vi "serial_connection_FSM_2.vi"(0 "commands_q":refnum<queue>, 5 "sensor_data_q":refnum<queue>, 11 "error in (no error)":errorcluster) -> (15 "error out":T1)   [LabVIEW 2019]
uses:
  arduino_FSM.ctl
  <vilib>/Instr/_visa.llb/VISA Configure Serial Port (Instr).vi
panel:
  out "Waveform Graph":dbl[](graph)
  in  "Arguments":string
  in  "VISA resource name out":refnum<visa-resource-name>
  out "Sampling Frequency":string="1"
  out "COM port":string="COM5"
  out "baud RATE":string="9600"
  in  "state_and_args":string
  out "Arduino FSM":T2
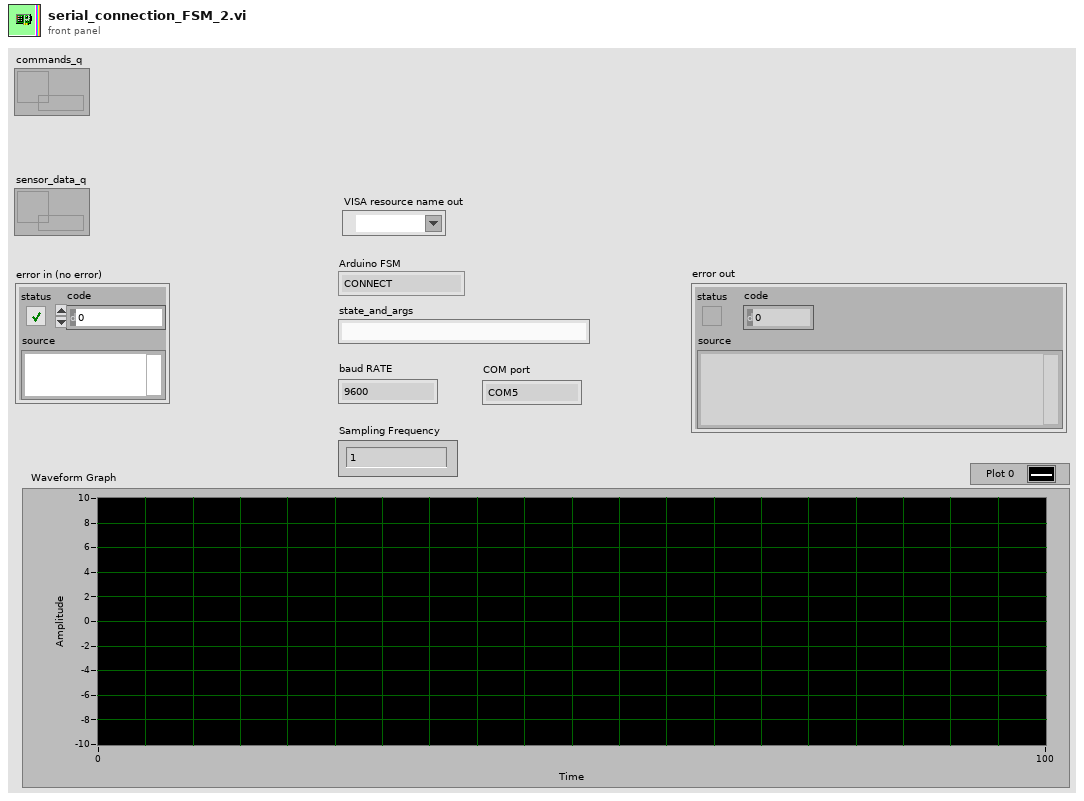
[diagram p1: front panel]
types:
  T1 = cluster{"status":bool, "code":u8, "source":string}
  T2 = typedef "arduino_FSM.ctl" = enum16{"CONNECT", "WAITING", "DISCONNECT", "READ", "WRITE", "WRONG_OP", "BYTE AVAIL?"}
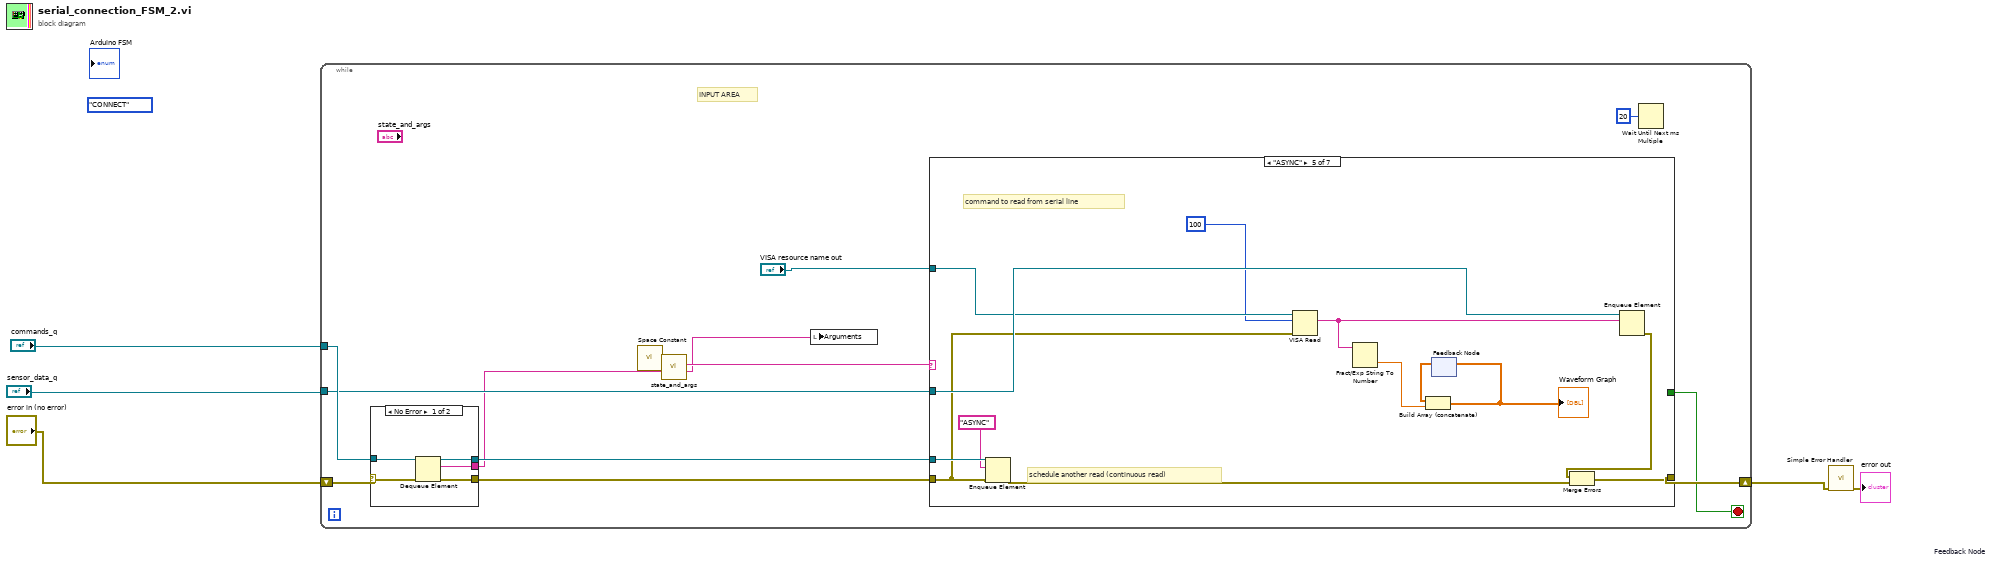
[diagram p0: block diagram]
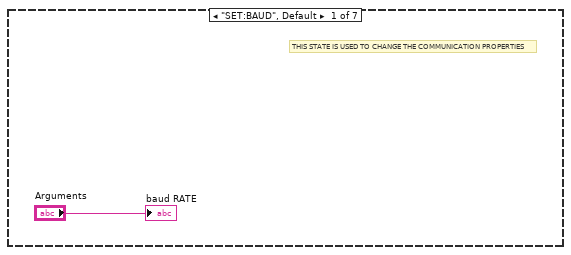
[diagram p2: hidden frame]
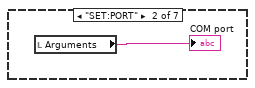
[diagram p3: hidden frame]
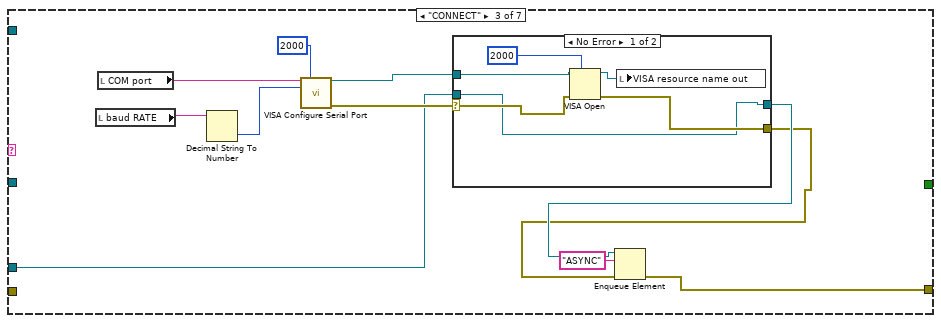
[diagram p4: hidden frame]
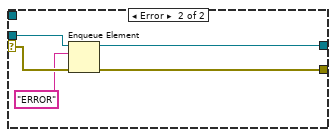
[diagram p5: hidden frame]
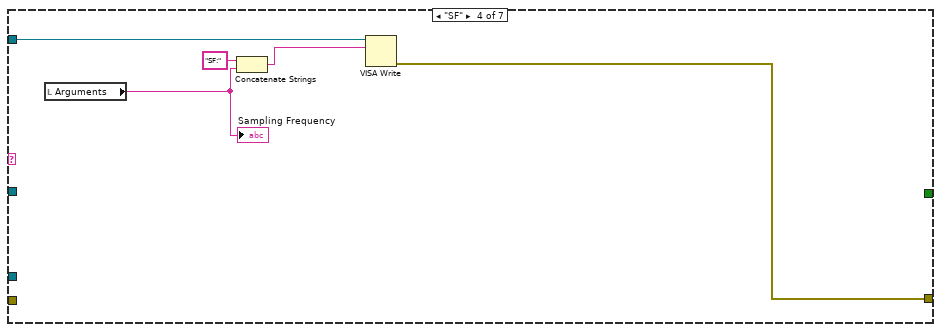
[diagram p6: hidden frame]
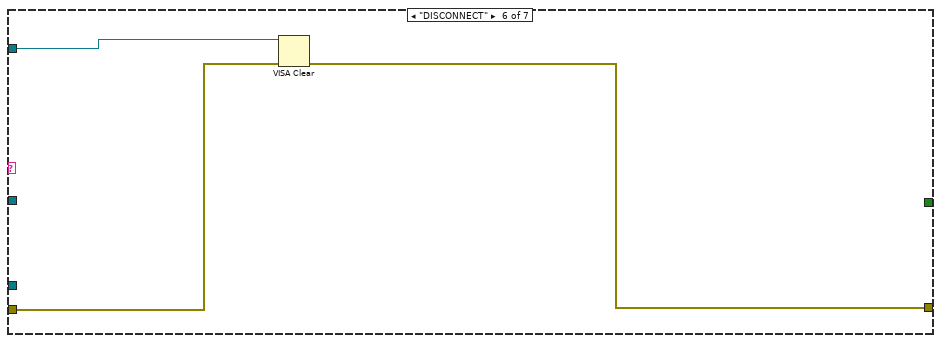
[diagram p7: hidden frame]
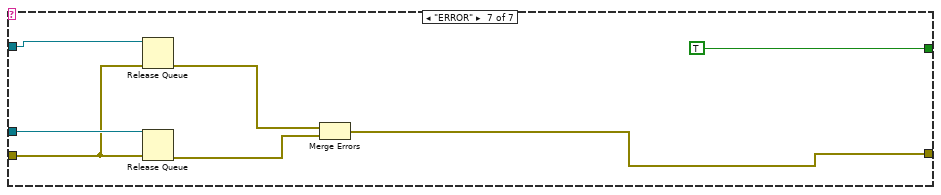
[diagram p8: hidden frame]
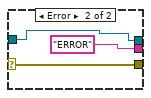
[diagram p9: hidden frame]
diagram:
  (unwired) arduino_FSM."CONNECT" ("Arduino FSM")
  n1 = while {
    tunnel: "commands_q" -> [w17]
    shift-right: [w14] -> w4
    shift-left: "error in (no error)" -> [w18]
    tunnel: "sensor_data_q" -> [w13]
    stop <- w12 stop-if-true
    # "INPUT AREA"
    n2 = case shown="No Error" w18 {
      selector: w18 -> [w75 w76]
      tunnel: w17 -> [w74 w77]
      tunnel: [w73 w77] -> w16
      tunnel: [w72 w76] -> w15
      tunnel: [w71 "ERROR"] -> w9
      frame No Error {
        n3 = Dequeue Element(queue=w74, error in (no error)=w75) -> (queue out=w73:refnum<queue>, element=w71:string, error out=w72:errorcluster)  [unwired: 1 in, 1 out]
      }
      frame Error {
      }
    }
    n4 = call <vilib>:"Space Constant.vi"() -> ("String"=w8:string)
    n5 = call "state_and_args.vi"("String"=w9, "DELIMITER (:)"=w8) -> ("Arguments"=w6:string, "State"=w7:string)  [unwired: 8 in]
    n6 = local write "Arguments"(w6) -> ()
    n7 = case shown="\"ASYNC\"" w7 {
      tunnel: w16 -> [_ _ w25 _ w60 _ w69]
      tunnel: w15 -> [_ _ _ _ w53 w63 w68]
      tunnel: [_ _ w21 w45 w58 w62 w65] -> w14
      tunnel: w13 -> [_ _ _ _ w56 _ w70]
      tunnel: [_ _ _ _ _ _ TRUE] -> w12
      tunnel: "VISA resource name out" -> [_ _ _ w44 w54 w61 _]
      frame "SET:BAUD", Default {
        # "THIS STATE IS USED TO CHANGE THE COMMUNICATION PROPERTIES"
        "baud RATE" <- "Arguments"
      }
      frame "SET:PORT" {
        n8 = local read "Arguments"() -> (→"COM port":string)
      }
      frame "CONNECT" {
        n9 = local read "baud RATE"() -> (w30:string)
        n10 = local read "COM port"() -> (w31:string)
        n11 = Decimal String To Number(string=w30) -> (number=w29:i32)  [unwired: 2 in, 1 out]
        n12 = call-poly "VISA Configure Serial Port"("VISA resource name"=w31, "timeout (10sec)"=u32 2000, "baud rate (9600)"=w29) -> ("VISA resource name out"=w27:refnum<visa-resource-name>, "error out"=w26:errorcluster)  [unwired: 11 in]
        n13 = case shown="No Error" w26 {
          selector: w26 -> [w36 w42]
          tunnel: w27 -> [w37 _]
          tunnel: w25 -> [w32 w41]
          tunnel: [w35 w39] -> w23
          tunnel: [w32 w38] -> w24
          frame No Error {
            n14 = VISA Open(timeout (0)=u32 2000 ("VISA Open timeout (0)"), error in (no error)=w36, VISA resource name=w37) -> (VISA resource name=w33:refnum<visa-resource-name>, error out=w35:errorcluster)  [unwired: 2 in]
            n15 = local write "VISA resource name out"(w33) -> ()
          }
          frame Error {
            n16 = Enqueue Element(queue=w41, element="ERROR", error in (no error)=w42) -> (queue out=w38:refnum<queue>, error out=w39:errorcluster)  [unwired: 1 in, 1 out]
          }
        }
        n17 = Enqueue Element(queue=w24, element="ASYNC", error in (no error)=w23) -> (error out=w21:errorcluster)  [unwired: 1 in, 2 out]
      }
      frame "SF" {
        n18 = local read "Arguments"() -> (w43:string)
        "Sampling Frequency" <- w43
        n19 = Concatenate Strings("SF:" ("string"), w43) -> (w46:string)
        n20 = VISA Write(VISA resource name=w44, write buffer=w46) -> (error out=w45:errorcluster)  [unwired: 1 in, 2 out]
      }
      frame "ASYNC" {
        # "command to read from serial line"
        # "schedule another read (continuous read)"
        n21 = Enqueue Element(queue=w60, element="ASYNC", error in (no error)=w53) -> (error out=w57:errorcluster)  [unwired: 1 in, 2 out]
        n22 = VISA Read(VISA resource name=w54, byte count=u32 100, error in (no error)=w53) -> (read buffer=w48:string)  [unwired: 3 out]
        n23 = Fract/Exp String To Number(string=w48) -> (number=w49:dbl)  [unwired: 3 in, 1 out]
        n24 = feedback #1 "Feedback Node"() -> (w51:dbl[])  [unwired: 1 in]
        n25 = Build Array (concatenate)(w51, w49) -> (w50:dbl[])
        "Waveform Graph" <- w50
        n26 = feedback-in #1(w50) -> ()
        n27 = Enqueue Element(queue=w56, element=w48) -> (error out=w55:errorcluster)  [unwired: 2 in, 2 out]
        n28 = Merge Errors(w55, w57) -> (w58:errorcluster)
      }
      frame "DISCONNECT" {
        n29 = VISA Clear(VISA resource name=w61, error in (no error)=w63) -> (error out=w62:errorcluster)  [unwired: 1 out]
      }
      frame "ERROR" {
        n30 = Release Queue(queue=w70, error in (no error)=w68) -> (error out=w67:errorcluster)  [unwired: 1 in, 2 out]
        n31 = Release Queue(queue=w69, error in (no error)=w68) -> (error out=w66:errorcluster)  [unwired: 1 in, 2 out]
        n32 = Merge Errors(w67, w66) -> (w65:errorcluster)
      }
    }
    n33 = Wait Until Next ms Multiple(millisecond multiple=u32 20) -> ()  [unwired: 1 out]
  }
  n34 = call <vilib>:"Simple Error Handler.vi"("error in (no error)"=w4) -> ("error out"=→"error out":errorcluster)  [unwired: 4 in, 4 out]
